vi "CPTR Adjust Update.vi"(0 "Register Buses":refnum<class "ni579x Register Bus v1 Host.lvclass">[](array[class]), 5 "cptr adjust distances":u16[](array[numeric]), 11 "error in":errorcluster, 12 "sync.cptr.period":u16=1) -> (4 "Register Buses (out)":refnum<class "ni579x Register Bus v1 Host.lvclass">[](array[class]), 15 "error out":errorcluster)   [LabVIEW 2012, in "ni579x Synchronization v1 Host.lvlib"]
doc: "Based on the input measurements, calculate and set the CPTR Adjust values on all the devices."
uses:
  <instrlib>/ni579x/Synchronization/v1/Host/ni579x Synchronization v1 Host.lvlib
  <instrlib>/ni579x/Register Bus/v1/Host/ni579x Register Bus v1 Host.lvclass
  <instrlib>/ni579x/Register Bus/v1/Host/Public/Register Read Request.ctl
  <instrlib>/ni579x/Synchronization/v1/Shared/ni579x Synchronization Register Addresses.ctl
  <instrlib>/ni579x/Config/v1/Shared/Types/ni579x Register Bus Subsystem ID.ctl
  <instrlib>/ni579x/Register Bus/v1/Host/Public/Register Write.ctl
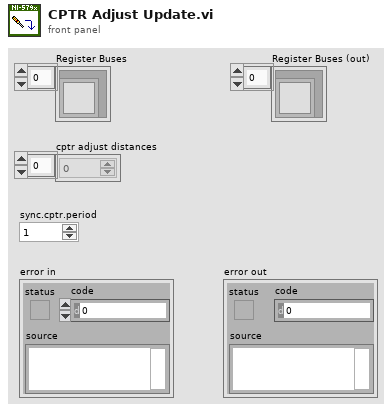
[diagram p1: front panel]
types:
  T1 = typedef "ni579x Register Bus Subsystem ID.ctl" = u8
  T2 = typedef "ni579x Synchronization Register Addresses.ctl" = enum16{"Signature", "Current Version", "Oldest Compatible Version", "Scratch Register", "sync.master", "sync.meas.enable", "sync.meas.ready", "sync.meas.arm", "sync.meas.valid", "sync.meas.value", "sync.cptr.adjust", "sync.cptr.period", "sync.meas.oversample factor"}
  T3 = typedef "ni579x Register Bus v1 Host.lvclass/Register Read Request.ctl" = cluster{"subsystem":u8, "address":u16}
  T4 = typedef "ni579x Register Bus v1 Host.lvclass/Register Write.ctl" = cluster{"subsystem":u8, "address":u16, "data":u32}
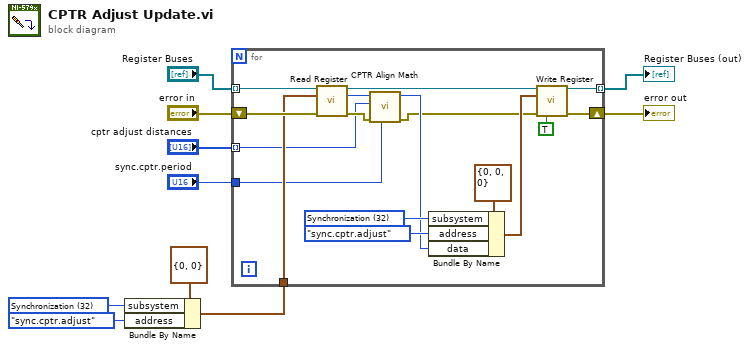
[diagram p0: block diagram]
diagram:
  w9 = T1 32 items=["FAM Register Operation"=0, "User Command"=16, "Synchronization"=32] ("Subsystem ID")
  n1 = Bundle By Name(cluster=T3 {"subsystem"=0, "address"=0} ("register read request"), "subsystem"=w9, "address"=ni579x_Synchronization_Register_Addresses."sync.cptr.adjust" ("Synchronization Registers")) -> (w6:T3)
  n2 = for {
    tunnel: [w16] -> w2 mode=indexing
    tunnel: "Register Buses" -> [w15] mode=indexing
    shift-right: [w17] -> w1
    shift-left: "error in" -> [w14]
    tunnel: w6 -> [w13]
    tunnel: "cptr adjust distances" -> [w11] mode=indexing
    tunnel: "sync.cptr.period" -> [w12]
    w25 = T1 32 items=["FAM Register Operation"=0, "User Command"=16, "Synchronization"=32] ("Subsystem ID")
    n3 = call <instrlib>:"Read Register.vi"("session in"=w15, "register read request"=w13, "error in"=w14) -> ("session out"=w19:refnum<class "ni579x Register Bus v1 Host.lvclass">, "data"=w22:u32, "error out"=w20:errorcluster)  [unwired: 10 in]
    n4 = call <instrlib>:"CPTR Align Math.vi"("sync.cptr.period"=w12, "error in"=w20, "measured cptr adjust distance"=w11, "sync.cptr.adjust"=w22) -> ("error out"=w18:errorcluster, "new cptr adjust"=w21:u16)  [unwired: 6 in]
    n5 = Bundle By Name(cluster=T4 {"subsystem"=0, "address"=0, "data"=0} ("register write"), "subsystem"=w25, "address"=ni579x_Synchronization_Register_Addresses."sync.cptr.adjust" ("Synchronization Registers"), "data"=w21) -> (w23:T4)
    n6 = call <instrlib>:"Write Register.vi"("session in"=w19, "register write"=w23, "error in"=w18, "wait until committed"=TRUE) -> ("session out"=w16:refnum<class "ni579x Register Bus v1 Host.lvclass">, "error out"=w17:errorcluster)  [unwired: 10 in]
  }
  "error out" <- w1
  "Register Buses (out)" <- w2
